vi "Init Core.vi"(0 "Display State In":T3, 5 "Path Overrides":T2, 7 "Environment Options":T1, 9 "Container State":T4, 11 "error in (no error)":errorcluster) -> (4 "Display State Out":T3, 15 "error out":errorcluster)   [LabVIEW 2020, in "WebView2 XControl.lvlib" / "WebView2 Control.xctl"]
uses:
  WebView2 Control.xctl
  <vilib>/_xctls/Container State.ctl
  State.ctl
  Webview2 Lib/WebView2 Control Object/WebView2 Control.lvclass
  Webview2 Lib/WebView2 Control Object/Paths.ctl
  Webview2 Lib/WebView2 Control Object/Core Env Options.ctl
  <vilib>/_xctls/XControlSupport.lvlib
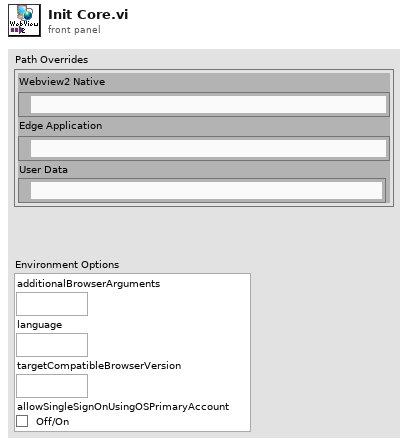
[diagram p1: front panel]
types:
  T1 = typedef "WebView2.lvlib/WebView2 Control.lvclass/Core Env Options.ctl" = cluster{"additionalBrowserArguments":string, "language":string, "targetCompatibleBrowserVersion":string, "allowSingleSignOnUsingOSPrimaryAccount":bool}
  T2 = typedef "WebView2.lvlib/WebView2 Control.lvclass/Paths.ctl" = cluster{"Webview2 Native":path, "Edge Application":path, "User Data":path}
  T3 = typedef "WebView2 XControl.lvlib/WebView2 Control.xctl/State.ctl" = cluster{"Control Object Ref":refnum<data-value>}
  T4 = typedef "XControlSupport.lvlib/Container State.ctl" = cluster{"Indicator?":bool, "Run Mode?":bool, " Refnum":refnum<vi>}
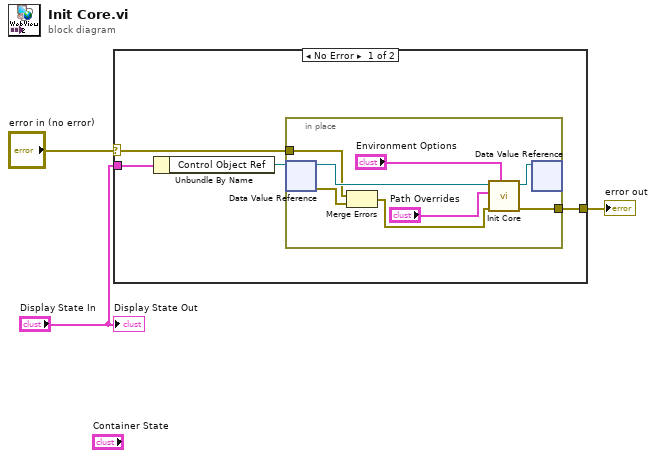
[diagram p0: block diagram]
diagram:
  n1 = case shown="No Error" "error in (no error)" {
    selector: "error in (no error)" -> [w6 w16]
    tunnel: [w5 w16] -> w2
    tunnel: "Display State In" -> [w4 _]
    frame No Error {
      n2 = Unbundle By Name(w4) -> ("Control Object Ref"=w7:refnum<data-value>)
      n3 = in-place {
        in-place-border: w6 -> [w14]
        in-place-border: [w13] -> w5
        n4 = in-place-dvr #1(w7) -> (w15:refnum<class "WebView2 Control.lvclass">, w8:errorcluster)
        n5 = Merge Errors(w14, w8) -> (w9:errorcluster)
        n6 = call "Init Core.vi"("Environment Options (Defaults)"="Environment Options", "error in (no error)"=w9, "Path Overrides (Empty=Default)"="Path Overrides", "WebView2 Control in"=w15) -> ("error out"=w13:errorcluster, "WebView2 Control out"=w10:refnum<class "WebView2 Control.lvclass">)  [unwired: 6 in]
        n7 = in-place-dvr #1(w10) -> ()  [unwired: 2 out]
      }
    }
    frame Error {
    }
  }
  "error out" <- w2
  "Display State Out" <- "Display State In"
